vi "Waveform_display.vi"(11 "error in (no error)":errorcluster) -> (1 "Waveform Chart":dbl(graph), 15 "error out":errorcluster)   [LabVIEW 2023, in "Task_1.lvlib"]
doc: "Display the waveform chart of the slider."
uses:
  Task_1.lvlib
  Control/Operations.ctl
  <vilib>/Utility/error.llb/DialogType.ctl
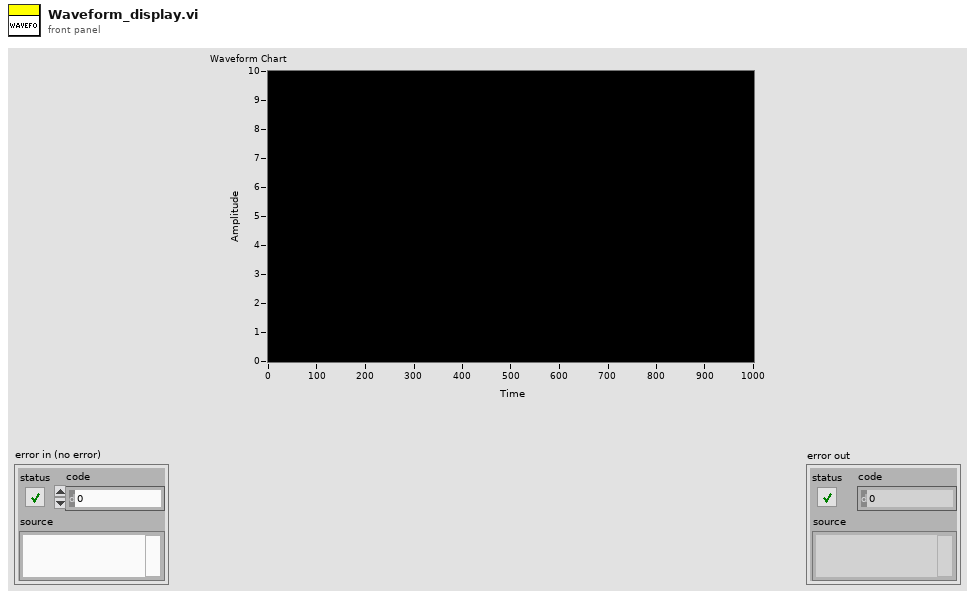
[diagram p1: front panel]
types:
  T1 = typedef "Task_1.lvlib/Operations.ctl" = enum16{"Create", "Gen_ref", "Generate", "Destroy"}
  T2 = typedef "DialogType.ctl" = u16
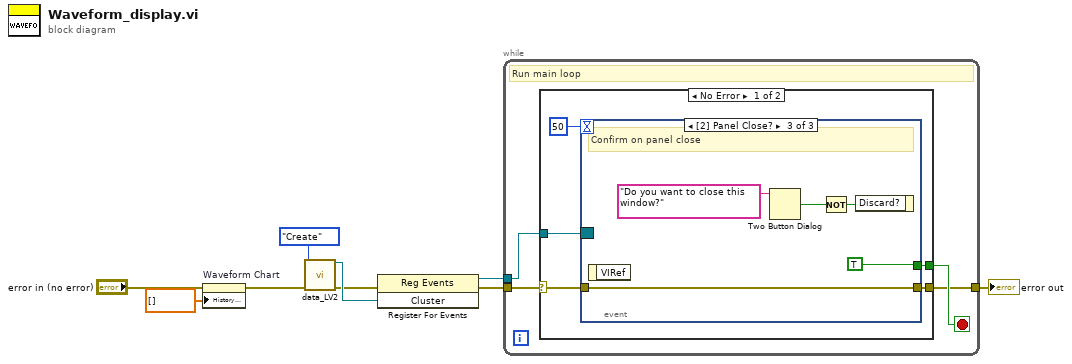
[diagram p0: block diagram]
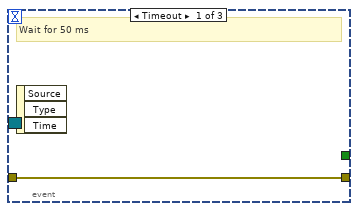
[diagram p2: hidden frame]
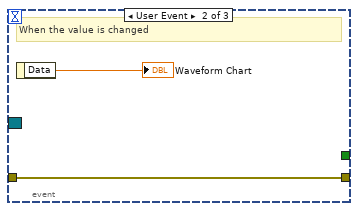
[diagram p3: hidden frame]
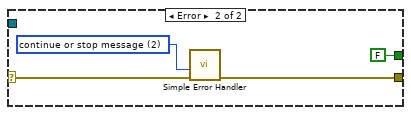
[diagram p4: hidden frame]
diagram:
  n1 = property on="Waveform Chart" class="WFChart (strict)"(error in="error in (no error)", "History Data"=dbl[] []) -> (error out=w3:errorcluster)  [unwired: 1 in, 1 out]
  n2 = call "data_LV2.vi"("Option"=Operations."Create", "error in (no error)"=w3) -> ("Cluster"=w9:refnum<user-event>, "error out"=w8:errorcluster)  [unwired: 12 in]
  n3 = register-events(error in=w8, w9) -> (reference out=w7:refnum<event-registration>, error out=w6:errorcluster)  [unwired: 1 in]
  n4 = while {
    tunnel: w7 -> [w13]
    tunnel: w6 -> [w12]
    tunnel: [w10] -> w1
    stop <- w11 stop-if-true
    # "Run main loop"
    n5 = case shown="No Error" w12 {
      selector: w12 -> [w16 w30]
      tunnel: w13 -> [w17 _]
      tunnel: [w15 FALSE] -> w11
      tunnel: [w14 w28] -> w10
      frame No Error {
        n6 = event shown="[2] Panel Close?" {
          selector: w17 -> [_ _ _]
          dyn-events: _ -> [_ _ _]
          timeout: 50 -> [_ _ _]
          tunnel: w16 -> [w19 w20 w25]
          tunnel: [_ _ TRUE] -> w15
          tunnel: [w19 w20 w25] -> w14
          event Timeout {
            # "Wait for 50 ms"
            n7 = event-data() -> ()  [unwired: 1 in, 3 out]
          }
          event User Event {
            # "When the value is changed"
            n8 = event-data() -> ("Data"=→"Waveform Chart":dbl)  [unwired: 1 in]
          }
          event Panel Close? {
            # "Confirm on panel close"
            n9 = event-data() -> ()  [unwired: 1 in, 1 out]
            n10 = Two Button Dialog(message="Do you want to close this window?") -> (T button?=w23:bool)  [unwired: 2 in]
            n11 = Not(x=w23) -> (.not. x?=w22:bool)
            n12 = event-data("Discard?"=w22) -> ()  [unwired: 1 in, 1 out]
          }
        }
      }
      frame Error {
        w27 = T2 2 items=["no dialog", "OK message", "continue or stop message", "OK message + warnings", "continue/stop + warnings"] ("type of dialog (OK msg:1)")
        n13 = call <vilib>:"Simple Error Handler.vi"("type of dialog (OK msg:1)"=w27, "error in (no error)"=w30) -> ("error out"=w28:errorcluster)  [unwired: 3 in, 4 out]
      }
    }
  }
  "error out" <- w1
